vi "open-loop_PID_tuner.vi"() -> ()   [LabVIEW 2009]
panel:
  out "Temperature [C]":dbl
  out "Elapsed Time":dbl
  out "Elapsed Time":dbl[](array[numeric])
  in  "RUN":bool
  in  "Reset":bool
  out "Measured Temperature":dbl[](array[numeric])
  out "Measured Current":dbl[](array[numeric])
  in  "End Program":bool
  out "Current Setopint":dbl[](array[numeric])
  in  "Save":bool
  out "Measured Current [A]":dbl
  out "Measured Voltage [V]":dbl
  out "Measured Current [A]":dbl(knob) scale=0.0..10.0
  out "Measured Voltage [V]":dbl(knob) scale=0.0..20.0
  in  "Current Setpoint [A]":dbl min=0.0 max=10.0
  in  "stop":bool
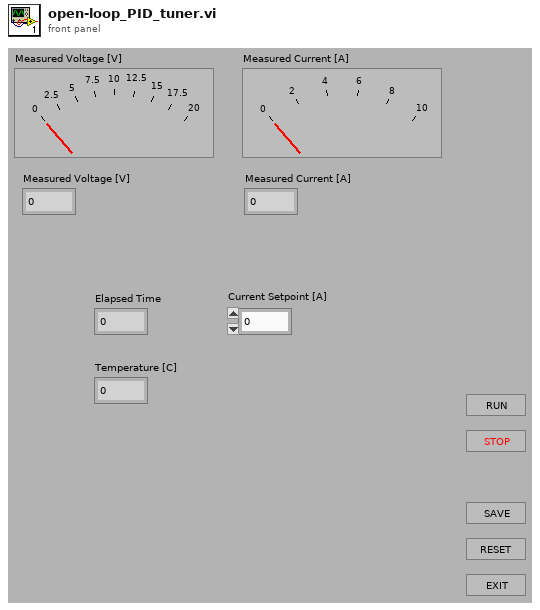
[diagram p1: front panel]
types:
  T1 = enum16{"open", "replace", "create", "open or create", "replace or create", "replace or create with confirmation"}
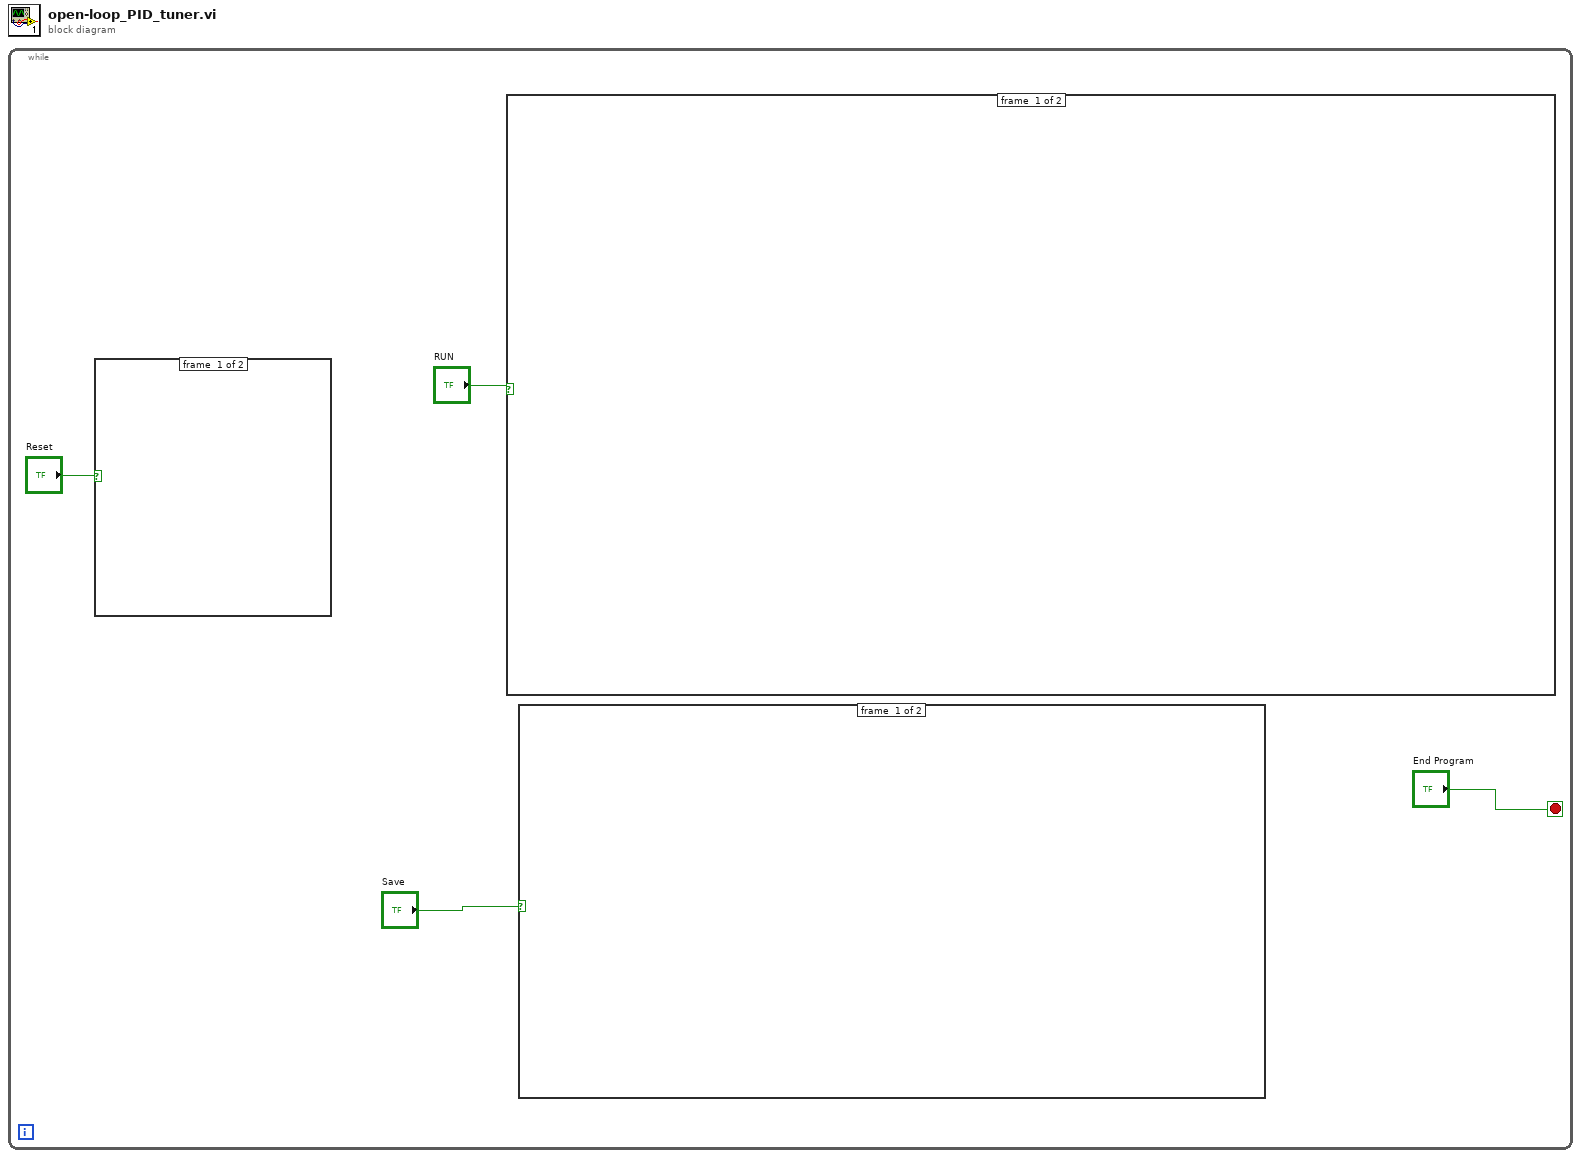
[diagram p0: block diagram]
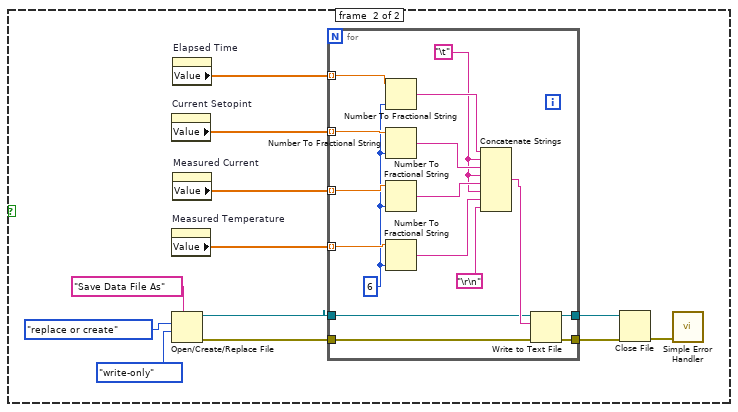
[diagram p2: hidden frame]
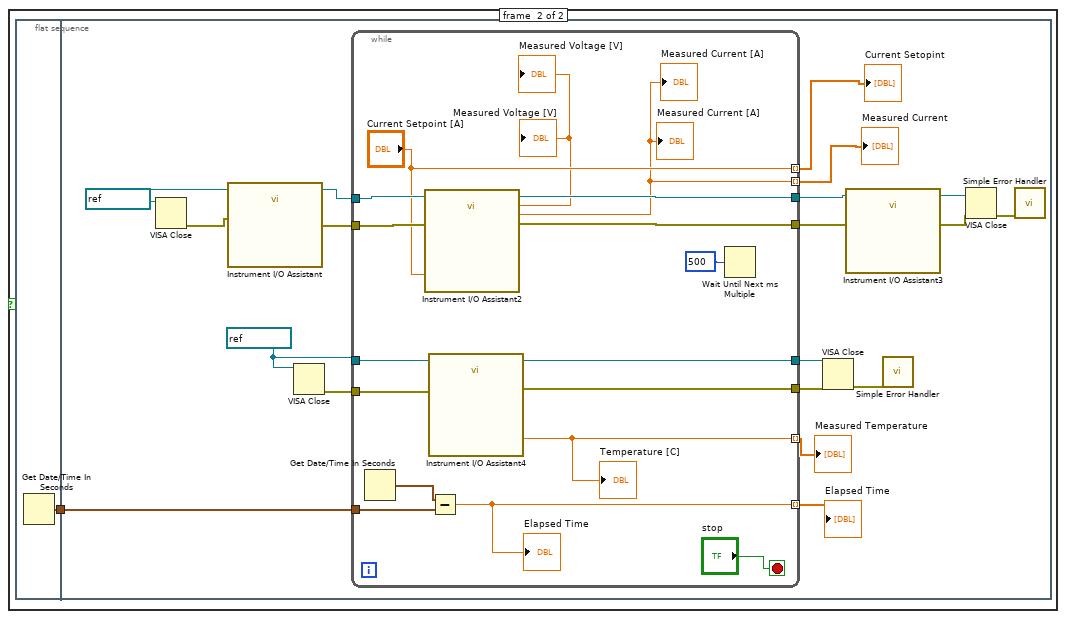
[diagram p3: hidden frame]
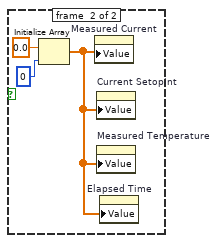
[diagram p4: hidden frame]
diagram:
  n1 = while {
    stop <- "End Program" stop-if-true
    n2 = case shown="True" "Reset" {
      frame #0 {
      }
      frame #1 {
        n3 = Initialize Array(0.0 ("element"), 0 ("dimension size")) -> (w71:dbl[])
        n4 = property on="Measured Current" class="Arr (strict)"("Value"=w71) -> ()  [unwired: 2 in, 2 out]
        n5 = property on="Current Setopint" class="Arr (strict)"("Value"=w71) -> ()  [unwired: 2 in, 2 out]
        n6 = property on="Measured Temperature" class="Arr (strict)"("Value"=w71) -> ()  [unwired: 2 in, 2 out]
        n7 = property on="Elapsed Time" class="Arr (strict)"("Value"=w71) -> ()  [unwired: 2 in, 2 out]
      }
    }
    n8 = case shown="True" "RUN" {
      frame #0 {
      }
      frame #1 {
        n9 = flat-sequence {
          tunnel: [w34] -> w33
          tunnel: w33 -> [w36]
          frame #0 {
            n10 = Get Date/Time In Seconds() -> (seconds since 1Jan1904=w34:timestamp)
          }
          frame #1 {
            w43 = refnum<visa-resource-name> "COM1" ("VISA resource name")
            w45 = refnum<visa-resource-name> "COM8" ("VISA resource name")
            n11 = VISA Close(VISA resource name=w45) -> (error out=w49:errorcluster)  [unwired: 1 in]
            n12 = call "Instrument I/O Assistant"("Session In"=w45, "error in"=w49) -> ("Session Out"=w53:refnum<visa-resource-name>, "error out"=w50:errorcluster)  [unwired: 24 in]
            n13 = VISA Close(VISA resource name=w43) -> (error out=w44:errorcluster)  [unwired: 1 in]
            n14 = while {
              tunnel: w53 -> [w69]
              tunnel: [w68] -> w52
              tunnel: [w67] -> w51
              tunnel: w50 -> [w66]
              tunnel: w44 -> [w64]
              tunnel: w43 -> [w63]
              tunnel: [w62] -> w42
              tunnel: [w61] -> w41
              tunnel: ["Current Setpoint [A]"] -> w39 mode=indexing
              tunnel: [w58] -> w38 mode=indexing
              tunnel: [w54] -> w37 mode=indexing
              tunnel: w36 -> [w57]
              tunnel: [w55] -> w35 mode=indexing
              stop <- "stop" stop-if-true
              n15 = Get Date/Time In Seconds() -> (seconds since 1Jan1904=w56:timestamp)
              n16 = call "Instrument I/O Assistant2"("Session In"=w69, "Current [A]"="Current Setpoint [A]", "error in"=w66) -> ("Session Out"=w68:refnum<visa-resource-name>, "Voltage"=→"Measured Voltage [V]" →"Measured Voltage [V]":dbl, "Current"=w58:dbl, "error out"=w67:errorcluster)  [unwired: 21 in]
              "Measured Current [A]" <- w58
              "Measured Current [A]" <- w58
              n17 = call "Instrument I/O Assistant4"("Session In"=w63, "error in"=w64) -> ("Session Out"=w62:refnum<visa-resource-name>, "Temperature [C]"=w54:dbl, "error out"=w61:errorcluster)  [unwired: 23 in]
              "Temperature [C]" <- w54
              n18 = Subtract(x=w56, y=w57) -> (x-y=w55:dbl)
              "Elapsed Time" <- w55
              n19 = Wait Until Next ms Multiple(millisecond multiple=u32 500) -> ()  [unwired: 1 out]
            }
            "Current Setopint" <- w39
            "Measured Current" <- w38
            "Measured Temperature" <- w37
            "Elapsed Time" <- w35
            n20 = VISA Close(VISA resource name=w42, error in (no error)=w41) -> (error out=w40:errorcluster)
            n21 = call "Instrument I/O Assistant3"("Session In"=w52, "error in"=w51) -> ("Session Out"=w48:refnum<visa-resource-name>, "error out"=w47:errorcluster)  [unwired: 24 in]
            n22 = call <vilib>:"Simple Error Handler.vi"("error in (no error)"=w40) -> ()  [unwired: 4 in, 5 out]
            n23 = VISA Close(VISA resource name=w48, error in (no error)=w47) -> (error out=w46:errorcluster)
            n24 = call <vilib>:"Simple Error Handler.vi"("error in (no error)"=w46) -> ()  [unwired: 4 in, 5 out]
          }
        }
      }
    }
    n25 = case shown="True" "Save" {
      frame #0 {
      }
      frame #1 {
        n26 = property on="Current Setopint" class="Arr (strict)"() -> ("Value"=w13:dbl[])  [unwired: 2 in, 2 out]
        n27 = property on="Measured Temperature" class="Arr (strict)"() -> ("Value"=w11:dbl[])  [unwired: 2 in, 2 out]
        n28 = Open/Create/Replace File(prompt="Save Data File As", operation (0:open)=T1."replace or create", access (0:read/write)=enum16{"read/write", "read-only", "write-only"}."write-only") -> (refnum out=w10:refnum<file>, error out=w9:errorcluster)  [unwired: 3 in, 1 out]
        n29 = property on="Elapsed Time" class="Arr (strict)"() -> ("Value"=w5:dbl[])  [unwired: 2 in, 2 out]
        n30 = property on="Measured Current" class="Arr (strict)"() -> ("Value"=w12:dbl[])  [unwired: 2 in, 2 out]
        n31 = for {
          tunnel: w13 -> [w32] mode=indexing
          tunnel: w12 -> [w31] mode=indexing
          tunnel: w11 -> [w30] mode=indexing
          tunnel: w10 -> [w24]
          tunnel: w9 -> [w23]
          tunnel: [w22] -> w8
          tunnel: [w21] -> w7
          tunnel: w5 -> [w19] mode=indexing
          w17 = "\t"
          w20 = i16 6 ("precision (6)")
          n32 = Number To Fractional String(number=w19, precision (6)=w20) -> (F-format string=w18:string)  [unwired: 2 in]
          n33 = Number To Fractional String(number=w32, precision (6)=w20) -> (F-format string=w29:string)  [unwired: 2 in]
          n34 = Number To Fractional String(number=w31, precision (6)=w20) -> (F-format string=w28:string)  [unwired: 2 in]
          n35 = Number To Fractional String(number=w30, precision (6)=w20) -> (F-format string=w27:string)  [unwired: 2 in]
          n36 = Concatenate Strings(w18, w17, w29, w17, w28, w17, w27, "\r\n") -> (w25:string)
          n37 = Write to Text File(file (use dialog)=w24, text=w25, error in=w23) -> (refnum out=w22:refnum<file>, error out=w21:errorcluster)  [unwired: 1 in, 1 out]
        }
        n38 = Close File(refnum=w8, error in=w7) -> (error out=w6:errorcluster)  [unwired: 1 out]
        n39 = call <vilib>:"Simple Error Handler.vi"("error in (no error)"=w6) -> ()  [unwired: 4 in, 5 out]
      }
    }
  }
